vi "Scale Compare.vi"(10 "Scale Position":string, 11 "Alliance Position":dbl) -> (3 "Scale Compare?":bool)   [LabVIEW 2017]
panel:
  # "SCALE COMPARE"
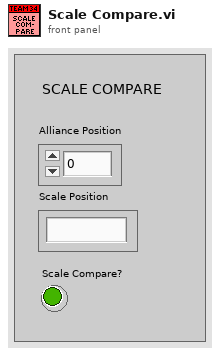
[diagram p1: front panel]
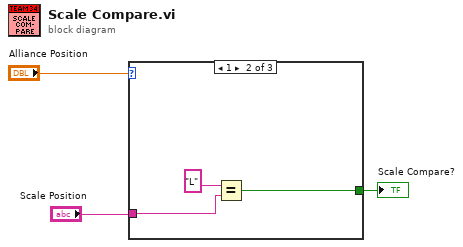
[diagram p0: block diagram]
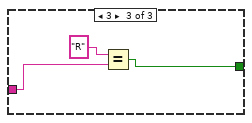
[diagram p3: hidden frame]
diagram:
  n1 = case shown="1" "Alliance Position" {
    tunnel: "Scale Position" -> [_ w6 w9]
    tunnel: [_ w4 w7] -> w2
    frame Default {
    }
    frame 1 {
      n2 = Equal?(x="L", y=w6) -> (x = y?=w4:bool)
    }
    frame 3 {
      n3 = Equal?(x="R", y=w9) -> (x = y?=w7:bool)
    }
  }
  "Scale Compare?" <- w2
